vi "loop_speed.vi"(9 "counter":i32, 10 "current time":u32, 11 "initial\ntime":u32) -> (2 "loop speed (Hz)":dbl, 3 "loop time (sec)":dbl)   [LabVIEW 2018]
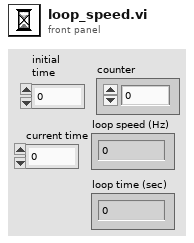
[diagram p1: front panel]
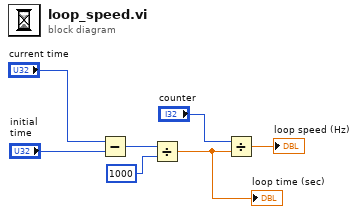
[diagram p0: block diagram]
diagram:
  n1 = Subtract(x="current time", y="initial\ntime") -> (x-y=w6:u32)
  n2 = Divide(x=w6, y=u32 1000) -> (x/y=w2:dbl)
  "loop time (sec)" <- w2
  n3 = Divide(x="counter", y=w2) -> (x/y=→"loop speed (Hz)":dbl)
